vi "Midi_main.vi"(11 "hub":string) -> ()   [LabVIEW 2022 SP3]
panel:
  in  "done":bool
  in  "Tab Control":T1(tab)
  in  "abort":bool
  in  "Test":bool
  in  "advertise":bool
  in  "Run":bool
  in  "note length (msec)":u8(slide)=104 scale=0.0..1000.0
  in  "Mapping formula":string="(sensor-40)/15+48"
  out "Converted note":string
  in  "Port":u16(ring) items=["A", "B", "C", "D", "E", "F"]
  in  "Sensor":u16(ring) items=["proximity", "light (color)", "light (reflected)", "force", "motor"]
  in  "BLE Name":string="something"
  out "current value":dbl(knob) scale=0.0..100.0
  in  "send":string
  in  "Read":bool
  out "sensor read":string
  out "Console":string
  out "Code":string
  out "running?":bool
  out "advertising":bool
  out "python good":bool
  out "error out":errorcluster
  out "ble?":bool
  # "1. Select your sensor and port\n2. Choose a BLE name and start advertising\n3. Connect on GarageBand (under settings/Advanced/Bluetooth )\n4.  Figure out your mapping formula\n5. Hit run"
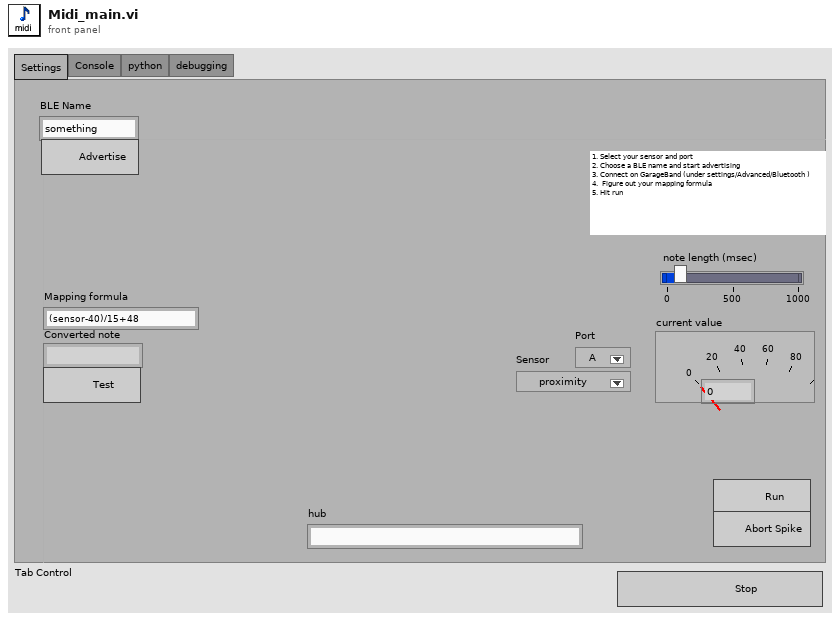
[diagram p1: front panel]
types:
  T1 = enum32{"Settings", "Console", "python", "debugging"}
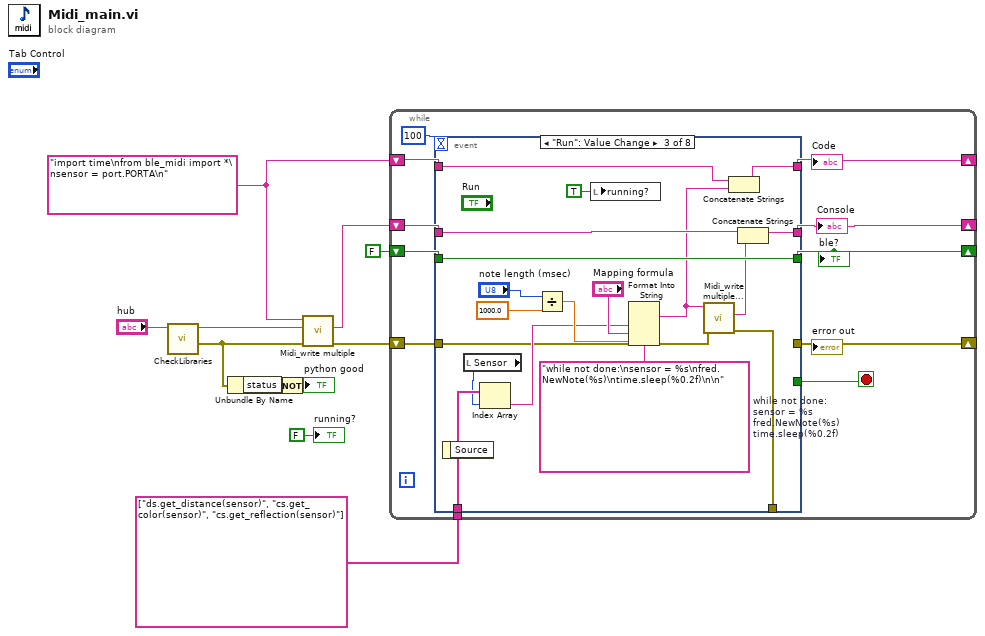
[diagram p0: block diagram]
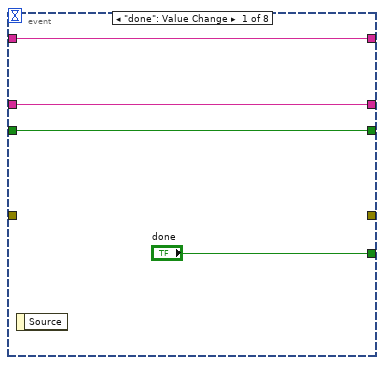
[diagram p2: hidden frame]
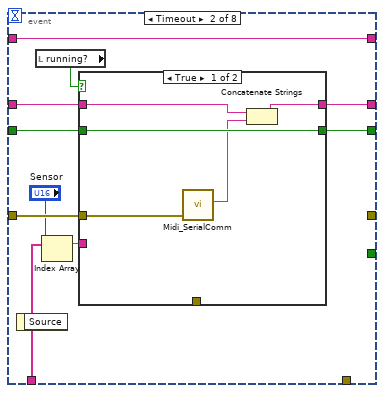
[diagram p3: hidden frame]
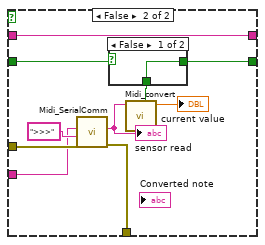
[diagram p4: hidden frame]
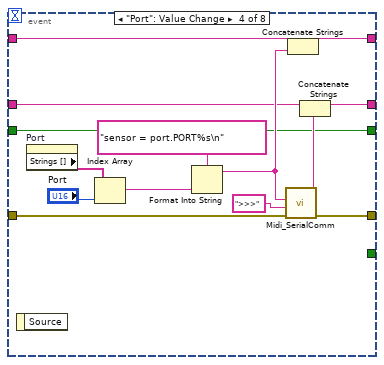
[diagram p6: hidden frame]
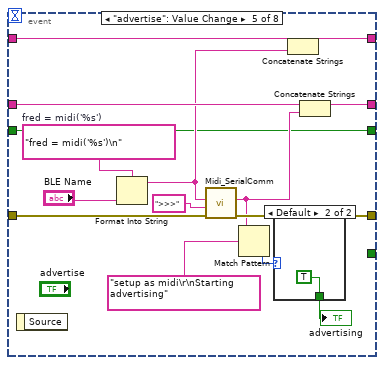
[diagram p7: hidden frame]
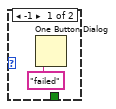
[diagram p8: hidden frame]
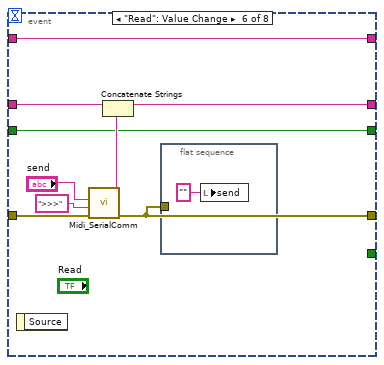
[diagram p9: hidden frame]
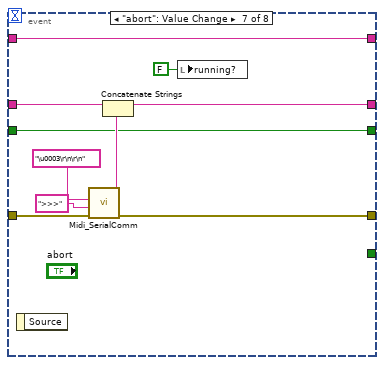
[diagram p10: hidden frame]
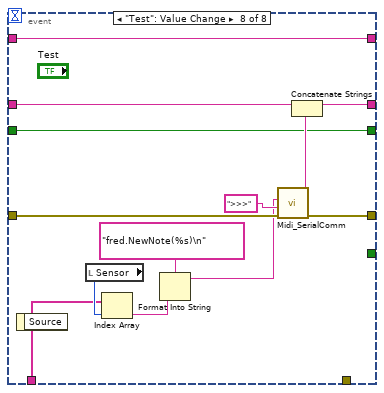
[diagram p11: hidden frame]
diagram:
  w4 = "import time\nfrom ble_midi import *\nsensor = port.PORTA\n"
  n1 = call "CheckLibraries.vi"("hub"="hub") -> ("error out"=w5:errorcluster, "console out"=w7:string)  [unwired: 9 in]
  n2 = Unbundle By Name(w5) -> ("status"=w10:bool)
  n3 = Not(x=w10) -> (.not. x?=→"python good":bool)
  n4 = call "Midi_write multiple.vi"("error in (no error)"=w5, "console in"=w7, "to write"=w4) -> ("error out"=w11:errorcluster, "console out"=w6:string)  [unwired: 7 in]
  n5 = while {
    shift-right: [w18] -> _
    shift-left: w6 -> [w19]
    shift-right: [w16] -> _
    shift-left: w4 -> [w17]
    shift-right: [w15] -> _
    shift-left: w11 -> [w22]
    shift-right: [w13] -> _
    shift-left: FALSE ("ble?") -> [w14]
    tunnel: string[] ["ds.get_distance(sensor)", "cs.get_color(sensor)", "cs.get_reflection(sensor)"] -> [w12]
    stop <- w21 stop-if-true
    n6 = event shown="[2] \"Run\": Value Change" {
      selector: _ -> [_ _ _ _ _ _ _ _]
      dyn-events: _ -> [_ _ _ _ _ _ _ _]
      timeout: 100 -> [_ _ _ _ _ _ _ _]
      tunnel: w22 -> [_ w36 w57 w80 w99 w110 w121 w134]
      tunnel: ["done" _ _ _ _ _ _ _] -> w21
      tunnel: w19 -> [w25 w35 w71 w75 w95 w109 w120 w133]
      tunnel: [w25 w34 w70 w73 w94 w107 w118 w131] -> w18
      tunnel: [w24 w33 w62 w76 w96 w106 w117 w130] -> w16
      tunnel: w17 -> [w24 w33 w63 w78 w97 w106 w117 w130]
      tunnel: [_ _ _ w79 w98 w104 w116 w129] -> w15
      tunnel: [w23 w32 w69 w72 w86 w103 w115 w128] -> w13
      tunnel: w14 -> [w23 w28 w69 w72 w86 w103 w115 w128]
      tunnel: w12 -> [_ w31 w61 _ _ _ _ w124]
      tunnel: [_ _ w54 _ _ _ _ _] -> _
      event "done": Value Change {
        n7 = event-data() -> ()  [unwired: 1 in, 1 out]
      }
      event Timeout {
        n8 = event-data() -> ()  [unwired: 1 in, 1 out]
        n9 = local read "running?"() -> (w27:bool)
        n10 = Index Array(array=w31, index="Sensor") -> (element=w29:string)
        n11 = case shown="True" w27 {
          tunnel: w36 -> [w40 w50]
          tunnel: w29 -> [_ w49]
          tunnel: w35 -> [w39 w46]
          tunnel: [w37 w46] -> w34
          tunnel: [_ w45] -> _
          tunnel: [w41 w44] -> w32
          tunnel: w28 -> [w41 w42]
          frame True {
            n12 = call "Midi_SerialComm.vi"("error in (no error)"=w40) -> ("read"=w38:string)  [unwired: 9 in, 1 out]
            n13 = Concatenate Strings(w39, w38) -> (w37:string)
          }
          frame False {
            n14 = call "Midi_SerialComm.vi"("error in (no error)"=w50, "wait for"=">>>", "To send"=w49) -> ("error out"=w45:errorcluster, "read"=w48:string)  [unwired: 7 in]
            "sensor read" <- w48
            n15 = call "Midi_convert.vi"("read"=w48) -> ("current value"=→"current value":dbl, "ble?"=w43:bool)  [unwired: 9 in]
            n16 = case shown="False" w42 {
              selector: w42 -> [_ w53]
              tunnel: [w52 w53] -> w44
              tunnel: w43 -> [w52 _]
              frame False {
              }
              frame True {
              }
            }
          }
        }
      }
      event "Run": Value Change {
        w64 = "while not done:\nsensor = %s\nfred.NewNote(%s)\ntime.sleep(%0.2f)\n\n"  # while not done: sensor = %s fred.NewNote(%s) time.sleep(%0.2f)
        n17 = event-data() -> ()  [unwired: 1 in, 1 out]
        n18 = local read "Sensor"() -> (w60:u16)
        n19 = Index Array(array=w61, index=w60) -> (element=w59:string)
        n20 = Divide(x="note length (msec)", y=1000.0) -> (x/y=w68:dbl)
        n21 = local write "running?"(TRUE ("running?")) -> ()
        n22 = Format Into String(format string=w64, w59, "Mapping formula", w68) -> (resulting string=w56:string)  [unwired: 2 in, 1 out]
        n23 = call "Midi_write multiple....vi"("error in (no error)"=w57, "to write"=w56) -> ("error out"=w54:errorcluster, "console out"=w55:string)  [unwired: 8 in]
        n24 = Concatenate Strings(w63, w56) -> (w62:string)
        n25 = Concatenate Strings(w71, w55) -> (w70:string)
      }
      event "Port": Value Change {
        n26 = event-data() -> ()  [unwired: 1 in, 1 out]
        n27 = property on="Port" class="Ring (strict)"() -> ("Strings []"=w83:string[])  [unwired: 2 in, 2 out]
        n28 = Index Array(array=w83, index="Port") -> (element=w85:string)
        n29 = Format Into String(format string="sensor = port.PORT%s\n", w85) -> (resulting string=w77:string)  [unwired: 2 in, 1 out]
        n30 = call "Midi_SerialComm.vi"("error in (no error)"=w80, "wait for"=">>>", "To send"=w77) -> ("error out"=w79:errorcluster, "read"=w74:string)  [unwired: 7 in]
        n31 = Concatenate Strings(w78, w77) -> (w76:string)
        n32 = Concatenate Strings(w75, w74) -> (w73:string)
      }
      event "advertise": Value Change {
        w92 = "fred = midi('%s')\n"  # fred = midi('%s')
        n33 = event-data() -> ()  [unwired: 1 in, 1 out]
        n34 = Format Into String(format string=w92, "BLE Name") -> (resulting string=w91:string)  [unwired: 2 in, 1 out]
        n35 = call "Midi_SerialComm.vi"("error in (no error)"=w99, "wait for"=">>>", "To send"=w91) -> ("error out"=w98:errorcluster, "read"=w90:string)  [unwired: 7 in]
        n36 = Match Pattern(string=w90, regular expression="setup as midi\r\nStarting advertising") -> (offset past match=w88:i32)  [unwired: 1 in, 3 out]
        n37 = case shown="Default" w88 {
          tunnel: [_ TRUE] -> w87
          frame -1 {
            n38 = One Button Dialog(message="failed") -> ()  [unwired: 1 in, 1 out]
          }
          frame Default {
          }
        }
        "advertising" <- w87
        n39 = Concatenate Strings(w97, w91) -> (w96:string)
        n40 = Concatenate Strings(w95, w90) -> (w94:string)
      }
      event "Read": Value Change {
        n41 = event-data() -> ()  [unwired: 1 in, 1 out]
        n42 = call "Midi_SerialComm.vi"("error in (no error)"=w110, "wait for"=">>>", "To send"="send") -> ("error out"=w104:errorcluster, "read"=w108:string)  [unwired: 7 in]
        n43 = Concatenate Strings(w109, w108) -> (w107:string)
        n44 = flat-sequence {
          tunnel: w104 -> [_]
          frame #0 {
            n45 = local write "send"("" ("send")) -> ()
          }
        }
      }
      event "abort": Value Change {
        n46 = event-data() -> ()  [unwired: 1 in, 1 out]
        n47 = call "Midi_SerialComm.vi"("error in (no error)"=w121, "wait for"=">>>", "To send"="\u0003\r\n\r\n" ("function name")) -> ("error out"=w116:errorcluster, "read"=w119:string)  [unwired: 7 in]
        n48 = Concatenate Strings(w120, w119) -> (w118:string)
        n49 = local write "running?"(FALSE ("running?")) -> ()
      }
      event "Test": Value Change {
        n50 = event-data() -> ()  [unwired: 1 in, 1 out]
        n51 = local read "Sensor"() -> (w125:u16)
        n52 = Index Array(array=w124, index=w125) -> (element=w123:string)
        n53 = Format Into String(format string="fred.NewNote(%s)\n", w123) -> (resulting string=w126:string)  [unwired: 2 in, 1 out]
        n54 = call "Midi_SerialComm.vi"("error in (no error)"=w134, "wait for"=">>>", "To send"=w126) -> ("error out"=w129:errorcluster, "read"=w132:string)  [unwired: 7 in]
        n55 = Concatenate Strings(w133, w132) -> (w131:string)
      }
    }
    "Console" <- w18
    "Code" <- w16
    "error out" <- w15
    "ble?" <- w13
  }
  "running?" <- FALSE ("running?")
